vi "TestHarnessWithSpoofedInput.vi"() -> ()   [LabVIEW 2015]
uses:
  QuadEnc/Output.ctl
  QuadEnc/Parameters.ctl
  <vilib>/Platform/TimedLoop/XDataNode/timing_clust.ctl
  <vilib>/Platform/TimedLoop/XDataNode/nitl_modes.ctl
  <vilib>/Platform/TimedLoop/XDataNode/wakeup.ctl
  <vilib>/rvi/DataTransferAndStorage/Container/Common/niFpgaContainerGetUniqueNameForEmu.vi
  <vilib>/rvi/DataTransferAndStorage/Container/Common/niFpgaContainerSetEmuInfo.vi
  <vilib>/rvi/eio/common/nirviEmuReportErrorAndStop.vi
  <vilib>/rvi/Emulation/niFpgaSctlEmulationGetInTimedLoop.vi
  <vilib>/rvi/Emulation/niFpgaEmulationReportErrorSimple.vi
  <vilib>/rvi/Emulation/niFpgaGetClockAttributes.vi
  <vilib>/rvi/Emulation/niFpgaCriticalErrorInLSC.vi
  <vilib>/rvi/DataTransferAndStorage/Container/Common/niFpgaContainerExecOnDevCompGetState.vi
  <vilib>/rvi/Emulation/niFpgaEmulationIsFPGAContextNoSignature.vi
  <vilib>/rvi/Memory/Memory_Emulation/niFpgaMemoryEmulationCacheClearOnFirstRun.vi
  <vilib>/rvi/Memory/Memory_Emulation/nirvimemoryEmulationManagerCache_MakeExclusive.vi
  <vilib>/rvi/Memory/Memory_Emulation/niFpgaMemoryEmulationValidateCache.vi
  <vilib>/rvi/Memory/Memory_Emulation/nirvimemoryEmulationManagerCache_InsertValue.vi
  <vilib>/Utility/error.llb/Clear Errors.vi
  <vilib>/rvi/Memory/Memory_Emulation/nirvimemoryEmulationManagerCache_ReleaseExclusive.vi
  <vilib>/rvi/Memory/Memory_Emulation/nirvimemoryEmulationManagerCache_GetValue.vi
  <vilib>/rvi/Memory/Memory_Emulation/nirvimemoryEmulationManagerCache_SetValue.vi
  <vilib>/rvi/Emulation/niFpgaProcessEmulError.vi
  <vilib>/rvi/LocalResourceManager/LocalResourceManager.xnode
  <vilib>/Platform/TimedLoop/XDataNode/XDataNode.xnode
  <vilib>/rvi/DataTransferAndStorage/Container/XNode/niFpgaContainer.xnode
  <vilib>/rvi/DataTransferAndStorage/Register/Emulation/niFpgaRegisterEmulationRefIn.vi
  <vilib>/Platform/TimedLoop/XDataNode/XDNodeRunTimeDep.lvlib
  QuadEnc/QuadEnc.lvlib
panel:
  out "Output":T1
  in  "spoofed tick rate":u32=20
  in  "spoofed ticks per rev":u32=10
  out "AbsPosition":i32
  out "RevPosition":i32
  in  "number of iterations":i32=20
  in  "ReversePolarity":bool
  in  "dTPerSec":sgl=10.0
  in  "RevPerPulse":sgl=0.001
  in  "dT":u32=4000000
  in  "done":bool
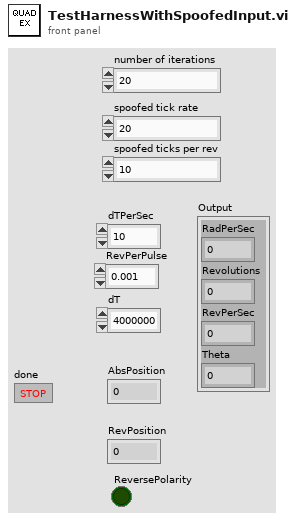
[diagram p1: front panel]
types:
  T1 = typedef "QuadEnc.lvlib/Output.ctl" = cluster{"RadPerSec":sgl, "Revolutions":sgl, "RevPerSec":sgl, "Theta":sgl}
  T2 = typedef "QuadEnc.lvlib/Parameters.ctl" = cluster{"ReversePolarity":refnum<k21>, "dTPerSec":refnum<k21>, "RevPerPulse":refnum<k21>, "dT":refnum<k21>}
  T3 = typedef "XDNodeRunTimeDep.lvlib/timing_clust.ctl" = cluster{"Expected End [f-1]":u64, "Actual End [f-1]":u64, "Finished Late? [f-1]":bool, "Expected End [i-1]":u64, "Actual End [i-1]":u64, "Finished Late? [i-1]":bool, "Expected Start [i]":u64, "Actual Start [i]":u64, "Expected Start [f]":u64, "Actual Start [f]":u64, "Source Name":string, "Structure Name":string, "Period":i64, "Deadline":i64, "Offset":i64, "Start":i64, "Priority":i32, "Timeout":i32, "Mode":T4, "Wakeup Reason":T5, "Error":errorcluster, "Source Type":string, "Secondary Source Type":string, "Global End Time":u64, "Global Start Time":u64, "Frame Duration":u64, "Iteration Duration":u64, "Assigned CPU":i32, "I/O Scan Engine Mode":u32}
  T4 = typedef "XDNodeRunTimeDep.lvlib/nitl_modes.ctl" = enum32{"No Change", "Process missed periods, maintain original phase", "Discard missed periods, maintain original phase", "Process missed periods, ignore original phase", "Discard missed periods, ignore original phase"}
  T5 = typedef "XDNodeRunTimeDep.lvlib/wakeup.ctl" = enum32{"Normal", "Aborted", "Asynchronous wakeup", "Timing source error", "Timed loop error", "Timeout"}
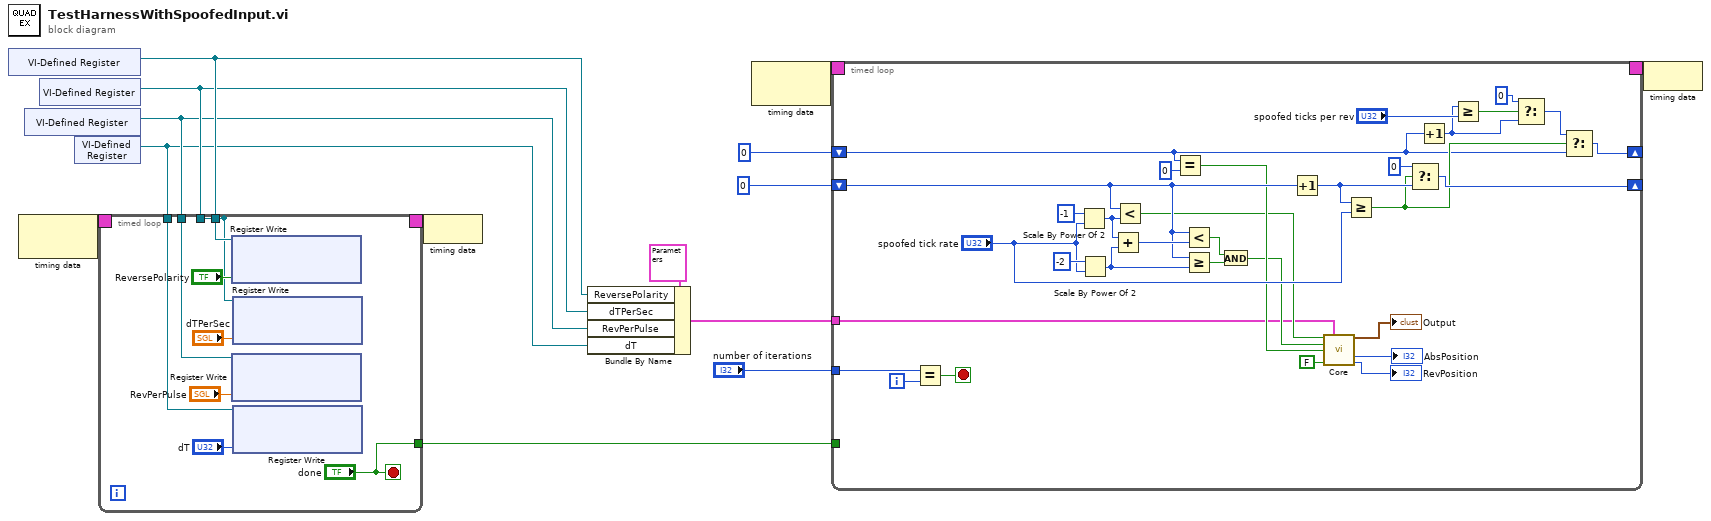
[diagram p0: block diagram]
diagram:
  n1 = xnode "VI-Defined Register"() -> ("Register Out"=w11:refnum<k21>)
  n2 = node-c288() -> (w14:T3)  [unwired: 1 in]
  n3 = xnode "VI-Defined Register"() -> ("Register Out"=w9:refnum<k21>)
  n4 = xnode "VI-Defined Register"() -> ("Register Out"=w10:refnum<k21>)
  n5 = xnode "VI-Defined Register"() -> ("Register Out"=w8:refnum<k21>)
  n6 = timed-loop {
    tunnel: w11 -> [w23]
    tunnel: [w21] -> _
    tunnel: w10 -> [w21]
    tunnel: w9 -> [w19]
    tunnel: w8 -> [w17]
    timing: w14 -> [_]
    timing-out: [_] -> w13
    tunnel: ["done"] -> w1
    stop <- "done" stop-if-true
    n7 = xnode ("Register Write")("Data"="ReversePolarity", "Register In"=w23) -> ()  [unwired: 1 out]
    n8 = xnode ("Register Write")("Data"="RevPerPulse", "Register In"=w19) -> ()  [unwired: 1 out]
    n9 = xnode ("Register Write")("Data"="dTPerSec", "Register In"=w21) -> ()  [unwired: 1 out]
    n10 = xnode ("Register Write")("Data"="dT", "Register In"=w17) -> ()  [unwired: 1 out]
  }
  n11 = node-c288(w13) -> ()
  n12 = Bundle By Name(cluster=T2 {"ReversePolarity"="ReversePolarity", "dTPerSec"="dTPerSec", "RevPerPulse"="RevPerPulse", "dT"="dT"} ("Parameters"), "ReversePolarity"=w11, "dTPerSec"=w10, "RevPerPulse"=w9, "dT"=w8) -> (w2:T2)
  n13 = node-c288() -> (w4:T3)  [unwired: 1 in]
  n14 = timed-loop {
    shift-right: [w46] -> _
    shift-left: u32 0 -> [w38]
    shift-right: [w45] -> _
    shift-left: u32 0 -> [w37]
    tunnel: "number of iterations" -> [w42]
    timing: w4 -> [_]
    timing-out: [_] -> w3
    tunnel: w2 -> [w27]
    tunnel: w1 -> [_]
    i -> [w41]
    stop <- w44 stop-if-true
    n15 = Equal?(x=w42, y=w41) -> (x = y?=w44:bool)
    n16 = Scale By Power Of 2(n=i16 -1, x="spoofed tick rate") -> (x*2^n=w54:u32)
    n17 = Scale By Power Of 2(n=i16 -2, x="spoofed tick rate") -> (x*2^n=w53:u32)
    n18 = Add(x=w54, y=w53) -> (x+y=w52:u32)
    n19 = Less?(x=w38, y=w54) -> (x < y?=w29:bool)
    n20 = Equal?(x=w37, y=u32 0) -> (x = y?=w30:bool)
    n21 = Less?(x=w38, y=w52) -> (x < y?=w51:bool)
    n22 = Greater Or Equal?(x=w38, y=w53) -> (x >= y?=w50:bool)
    n23 = And(x=w51, y=w50) -> (x .and. y?=w28:bool)
    n24 = Increment(x=w38) -> (x+1=w47:u32)
    n25 = call "Core.vi"("A"=w29, "Parameters"=w27, "B"=w28, "Z"=w30, "reset"=FALSE) -> ("Output"=→"Output":T1, "AbsPosition"=→"AbsPosition":i32, "RevPosition"=→"RevPosition":i32)  [unwired: 7 in, 1 out]
    n26 = Greater Or Equal?(x=w47, y="spoofed tick rate") -> (x >= y?=w39:bool)
    n27 = Select(t=u32 0, s=w39, f=w47) -> (s? t:f=w46:u32)
    n28 = Increment(x=w37) -> (x+1=w35:u32)
    n29 = Greater Or Equal?(x=w35, y="spoofed ticks per rev") -> (x >= y?=w36:bool)
    n30 = Select(t=u32 0 ("s? t:f"), s=w36, f=w35) -> (s? t:f=w34:u32)
    n31 = Select(t=w34, s=w39, f=w37) -> (s? t:f=w45:u32)
  }
  n32 = node-c288(w3) -> ()
